vi "se_main.vi"(6 "se.mot.p.target":cluster{"x":fxp<+/-,16,1>, "y":fxp<+/-,16,1>}, 8 "outputParams":T4, 9 "se.p.modes":T6, 10 "se.p.durationTrigger":u16=100, 11 "scanClocks":T7={"se.mot.p.clocks"={"moveToDecFactor"=0, "moveToWaveSize"=0, "se.mot.p.invDec"=0.0}, "se.p.clocks"={"outputRate"=0, "fastDecFactor"=0, "outWaveSizeFast"=0, "pplUpsampling"=0, "numLines"=0, "se.p.fastInvDec"=0.0, "se.p.slowUpStep"=0.0, "se.p.outWaveSizeSlow"=0, "blankingMax"=0, "se.p.fastBlanking"={"startFwd"=0, "endFwd"=0, "startBwd"=0, "endBwd"=0, "disableBlanking"=FALSE, "useCoarseCounter"=TRUE}}}) -> (0 "clocksOut":T3, 1 "se.o.position":T2 {"outputInt"."x" format="%.16g"; "outputInt"."y" format="%.16g"}, 2 "se.mot.s.origin":T5, 3 "se.mot.s.running":bool, 4 "indices":T1, 5 "debug":cluster{"blanking":u32, "pixelEvent":bool}, 7 "se.s.blankingOff":bool)   [LabVIEW 2016]
uses:
  <vilib>/rvi/Emulation/niFpgaEmulationIsFPGAContextNoSignature.vi
  <vilib>/rvi/Emulation/niFpgaSctlEmulationGetInTimedLoop.vi
  <vilib>/rvi/errors/niFpgaSetErrorForExecOnDevCompSimple.vi
  <vilib>/rvi/eio/common/nirviEmuReportErrorAndStop.vi
  <vilib>/rvi/DataTransferAndStorage/Container/Common/niFpgaContainerGetUniqueNameForEmu.vi
  <vilib>/rvi/FIFO/Fifo_Resource/nirvififoEmulationSetSize.vi
  <vilib>/rvi/FIFO/Fifo_Resource/nirviFifoEmulationQueueMgr.vi
  <instcachedir>/0/nirviFifoEmulationQueueMgr_E5CAEC123FF24DC58D834DCA3CDAA9B5.lvgen/nirviFifoEmulationQueueMgr_E5CAEC123FF24DC58D834DCA3CDAA9B5_010.vi
  <vilib>/rvi/FIFO/Fifo_Resource/nirvififoEmulationDetermineInputValidOut.vi
  <vilib>/rvi/FIFO/Fifo_Resource/nirvififoEmulationCreateLock.vi
  <vilib>/rvi/Emulation/niFpgaProcessEmulError.vi
  <vilib>/rvi/FIFO/Fifo_Resource/nirvififoEmulationObtainLock.vi
  <vilib>/rvi/FIFO/Fifo_Resource/nirvififoEmulationReleaseLock.vi
  <vilib>/rvi/occurrence/nirviWaitOnOccurrenceBase.vi
  <vilib>/rvi/errors/nirviReportUnexpectedCaseInternalError.vi
  <vilib>/rvi/errors/nirviReportUnexpectedCaseInternalError (U32).vi
  <vilib>/rvi/Memory/Memory_Emulation/niFpgaMemoryEmulationCacheClearOnFirstRun.vi
  <vilib>/rvi/Memory/Memory_Emulation/nirvimemoryEmulationManagerCache_MakeExclusive.vi
  <vilib>/rvi/Memory/Memory_Emulation/niFpgaMemoryEmulationValidateCache.vi
  <vilib>/rvi/Memory/Memory_Emulation/nirvimemoryEmulationManagerCache_InsertValue.vi
  <vilib>/Utility/error.llb/Clear Errors.vi
  <vilib>/rvi/Memory/Memory_Emulation/nirvimemoryEmulationManagerCache_ReleaseExclusive.vi
  <vilib>/rvi/Memory/Memory_Emulation/nirvimemoryEmulationManagerCache_GetValue.vi
  <vilib>/rvi/Memory/Memory_Emulation/nirvimemoryEmulationManagerCache_SetValue.vi
  <vilib>/rvi/DataTransferAndStorage/Container/XNode/niFpgaContainer.xnode
  <vilib>/rvi/FIFO/Fifo_Resource/nirvififoEmulationWrite.vi
  <vilib>/rvi/DataTransferAndStorage/Register/Emulation/niFpgaRegisterEmulation.vi
  <vilib>/rvi/FXPMathLib/FxpInterpret/XNode/nifxpmath_Interpret.xnode
  <instrlib>/_niInstr/Basic Elements/v1/FPGA/niInstr Basic Elements v1 FPGA.lvlib
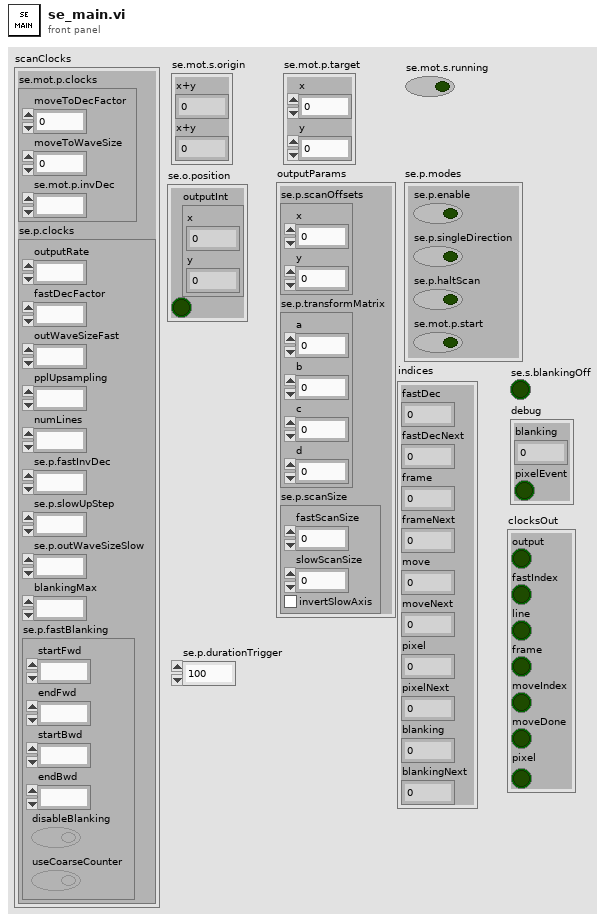
[diagram p1: front panel]
types:
  T1 = cluster{"fastDec":u16, "fastDecNext":u16, "frame":u16, "frameNext":u16, "move":u16, "moveNext":u16, "pixel":u16, "pixelNext":u16, "blanking":u32, "blankingNext":u32}
  T2 = cluster{"outputInt":cluster{"y":fxp<+/-,16,1>, "y":fxp<+/-,16,1>}, bool}
  T3 = cluster{"output":bool, "fastIndex":bool, "line":bool, "frame":bool, "moveIndex":bool, "moveDone":bool, "pixel":bool}
  T4 = cluster{"se.p.scanOffsets":cluster{"x":fxp<+/-,16,1>, "y":fxp<+/-,16,1>}, "se.p.transformMatrix":cluster{"a":fxp<+/-,18,2>, "b":fxp<+/-,18,2>, "c":fxp<+/-,18,2>, "d":fxp<+/-,18,2>}, "se.p.scanSize":cluster{"fastScanSize":fxp<+,17,1>, "slowScanSize":fxp<+,17,1>, "invertSlowAxis":bool}}
  T5 = cluster{"x+y":fxp<+/-,18,2>, "x+y":fxp<+/-,18,2>}
  T6 = cluster{"se.p.enable":bool, "se.p.singleDirection":bool, "se.p.haltScan":bool, "se.mot.p.start":bool}
  T7 = cluster{"se.mot.p.clocks":cluster{"moveToDecFactor":u16, "moveToWaveSize":u16, "se.mot.p.invDec":fxp<+,16,0>}, "se.p.clocks":cluster{"outputRate":u16, "fastDecFactor":u16, "outWaveSizeFast":u16, "pplUpsampling":u16, "numLines":u16, "se.p.fastInvDec":fxp<+,22,0>, "se.p.slowUpStep":fxp<+,28,0>, "se.p.outWaveSizeSlow":u16, "blankingMax":u32, "se.p.fastBlanking":cluster{"startFwd":u32, "endFwd":u32, "startBwd":u32, "endBwd":u32, "disableBlanking":bool, "useCoarseCounter":bool}}}
  T8 = cluster{"moveToDecFactor":u16, "moveToWaveSize":u16, "se.mot.p.invDec":fxp<+,16,0>}
  T9 = cluster{"outputRate":u16, "fastDecFactor":u16, "outWaveSizeFast":u16, "pplUpsampling":u16, "numLines":u16, "se.p.fastInvDec":fxp<+,22,0>, "se.p.slowUpStep":fxp<+,28,0>, "se.p.outWaveSizeSlow":u16, "blankingMax":u32, "se.p.fastBlanking":cluster{"startFwd":u32, "endFwd":u32, "startBwd":u32, "endBwd":u32, "disableBlanking":bool, "useCoarseCounter":bool}}
  T10 = cluster{"startFwd":u32, "endFwd":u32, "startBwd":u32, "endBwd":u32, "disableBlanking":bool, "useCoarseCounter":bool}
  T11 = cluster{"index":u16, "next":u16, "blanking":u32, "blankingNext":u32}
  T12 = cluster{"interpOutput":fxp<+/-,19,2>, "interpOutput":fxp<+/-,19,2>}
  T13 = cluster{"a":fxp<+/-,18,2>, "b":fxp<+/-,18,2>, "c":fxp<+/-,18,2>, "d":fxp<+/-,18,2>}
  T14 = cluster{"fastScanSize":fxp<+,17,1>, "slowScanSize":fxp<+,17,1>, "invertSlowAxis":bool}
  T15 = cluster{"se.p.scanOffsets":cluster{"x":bool, "y":bool}, "se.p.transformMatrix":cluster{"a":bool, "b":bool, "c":bool, "d":bool}, "se.p.scanSize":cluster{"fastScanSize":bool, "slowScanSize":bool, "invertSlowAxis":bool}}
  T16 = cluster{"xOut":fxp<+/-,18,2>, "yOut":fxp<+/-,18,2>}
  T17 = cluster{"fastScanSize":bool, "slowScanSize":bool, "invertSlowAxis":bool}
  T18 = cluster{cluster{"y":fxp<+/-,16,1>, "y":fxp<+/-,16,1>}, bool}
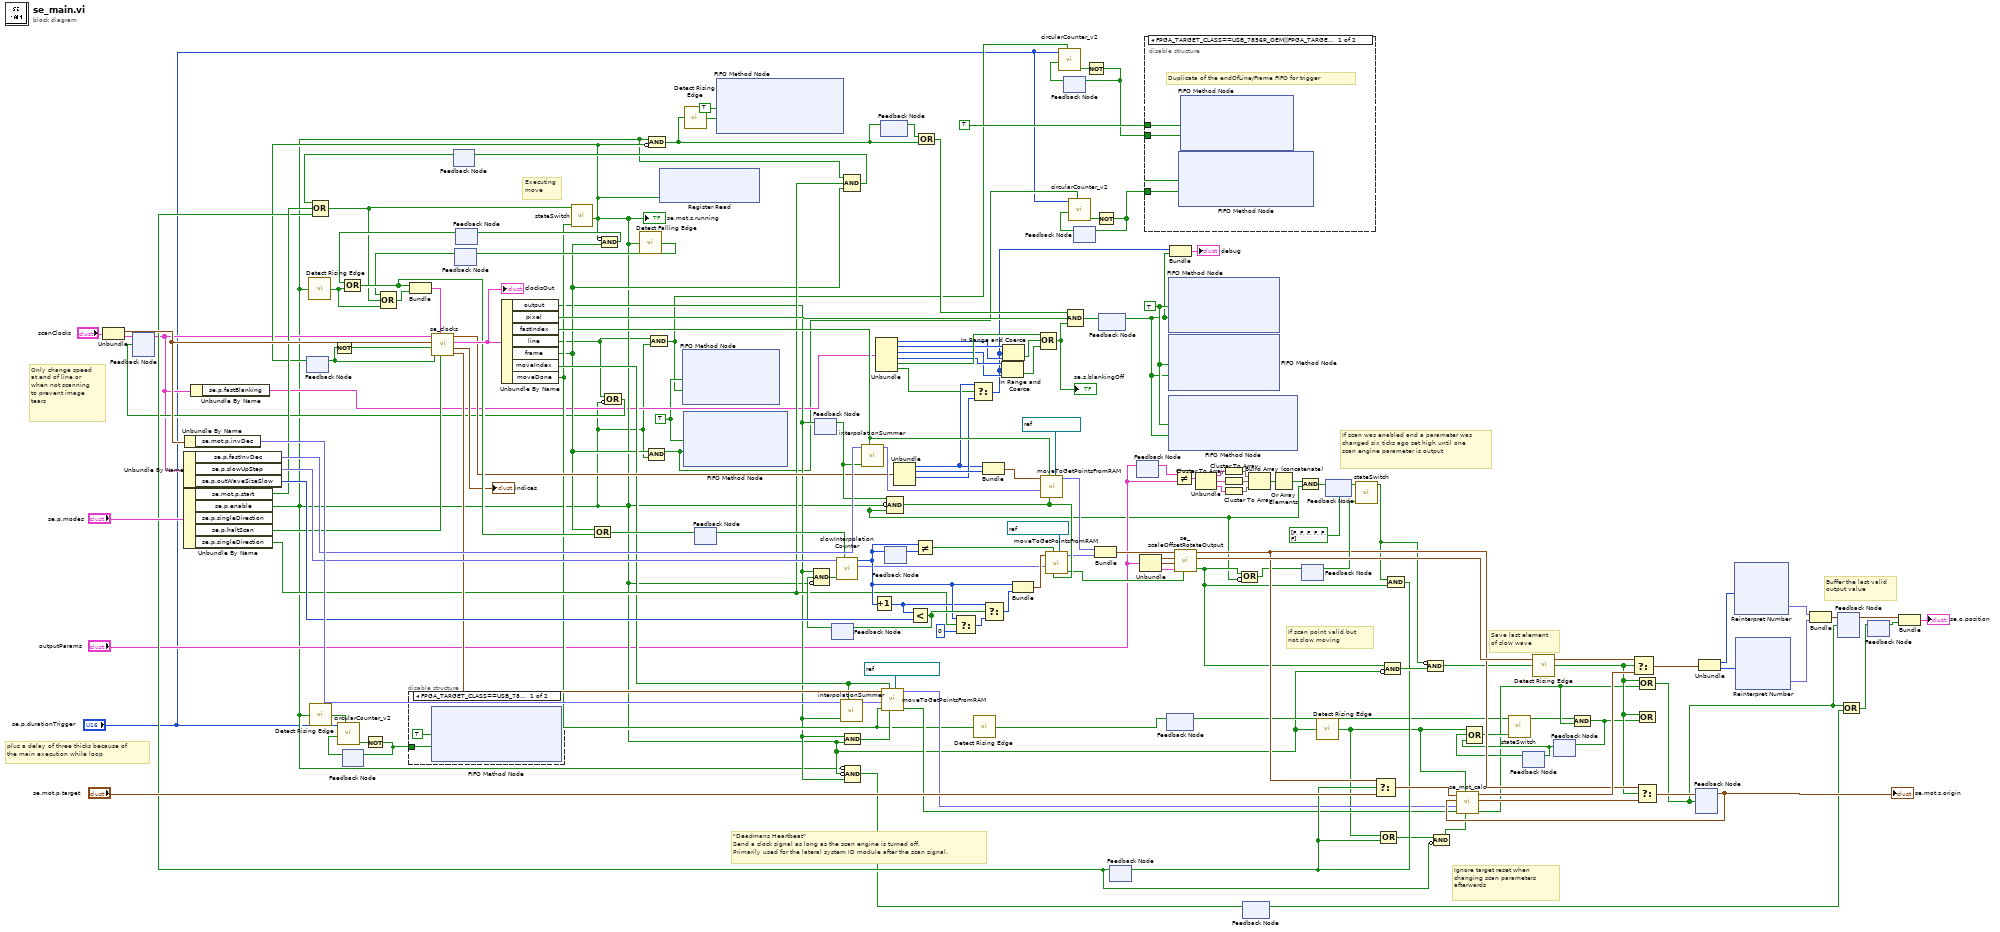
[diagram p0: block diagram]
diagram:
  w2 = TRUE ("Element")
  w20 = TRUE ("Element")
  # "plus a delay of three thicks because of\nthe main execution while loop"
  # "Only change speed at end of line or when not scanning to prevent image tears"
  # "Buffer the last valid output value"
  # "\"Deadmans Heartbeat\"\nSend a clock signal as long as the scan engine is turned off.\nPrimarily used for the lateral system ID module after the scan signal."
  # "Ignore target reset when changing scan parameters afterwards"
  # "If scan point valid but not slow moving"
  # "If scan was enabled and a parameter was changed six ticks ago set high until one scan engine parameter is output"
  # "Save last element \nof slow wave"
  # "Executing\nmove"
  n1 = Unbundle("scanClocks") -> ("se.mot.p.clocks"=w164:T8, "se.p.clocks"=w25:T9)
  n2 = feedback #1() -> (w24:T9)  [unwired: 1 in]
  n3 = Unbundle By Name(w24) -> ("se.p.fastInvDec"=w159:fxp<+,22,0>, "se.p.slowUpStep"=w160:fxp<+,28,0>, "se.p.outWaveSizeSlow"=w161:u16)
  n4 = Unbundle By Name("se.p.modes") -> ("se.mot.p.start"=w76:bool, "se.p.enable"=w14:bool, "se.p.haltScan"=w158:bool, "se.p.singleDirection"=w75:bool)  [unwired: 1 out]
  n5 = Unbundle By Name(w164) -> ("se.mot.p.invDec"=w162:fxp<+,16,0>)
  n6 = Unbundle By Name(w24) -> ("se.p.fastBlanking"=w26:T10)
  n7 = feedback #2() -> (w131:bool)  [unwired: 1 in]
  n8 = call <instrlib>:"Detect Rising Edge.vi"("signal"=w14) -> ("edge detected"=w74:bool)  [unwired: 14 in]
  n9 = call <instrlib>:"Detect Rising Edge.vi"("signal"=w14) -> ("edge detected"=w17:bool)  [unwired: 14 in]
  n10 = Not(x=w131) -> (.not. x?=w132:bool)
  n11 = feedback #3() -> (w15:bool)  [unwired: 1 in]
  n12 = call "circularCounter_v2.vi"("reset"=w17, "doStep"=w15, "maxCount"="se.p.durationTrigger") -> ("maxReached"=w18:bool)  [unwired: 5 in, 3 out]
  n13 = Not(x=w18) -> (.not. x?=w16:bool)
  n14 = feedback-in #3(w16) -> ()
  n15 = disable-structure shown="FPGA_TARGET_CLASS==USB_7856R_OEM||FPGA_TARGET_CLASS==USB_7856R" {
    disable-tunnel: w16 -> [w165 _]
    frame condition #0 (active) {
      n16 = xnode ("FIFO Method Node")("Element"=TRUE, "Input Valid"=w165) -> ()  [unwired: 1 in, 2 out]
    }
    frame condition #1 {
    }
  }
  n17 = feedback #4() -> (w127:bool)  [unwired: 1 in]
  n18 = feedback #5() -> (w72:bool)  [unwired: 1 in]
  n19 = feedback #6() -> (w124:bool)  [unwired: 1 in]
  n20 = Compound Arithmetic op=OR(w124, w74) -> (w91:bool)
  n21 = feedback #7() -> (w136:bool)  [unwired: 1 in]
  n22 = feedback #8() -> (w137:bool)  [unwired: 1 in]
  n23 = feedback #9() -> (w135:bool)  [unwired: 1 in]
  n24 = Unbundle(w26) -> ("startFwd"=w143:u32, "endFwd"=w144:u32, "startBwd"=w145:u32, "endBwd"=w146:u32, "disableBlanking"=w149:bool, "useCoarseCounter"=w64:bool)
  n25 = feedback #10() -> (w139:bool)  [unwired: 1 in]
  n26 = feedback #11() -> (w121:u16)  [unwired: 1 in]
  n27 = feedback #12() -> (w13:bool)  [unwired: 1 in]
  n28 = feedback #13() -> (w8:bool)  [unwired: 1 in]
  n29 = feedback #14() -> (w1:bool)  [unwired: 1 in]
  n30 = feedback #15() -> (w45:bool)  [unwired: 1 in]
  n31 = Compound Arithmetic op=OR(w127, w76, w45) -> (w73:bool)
  n32 = Compound Arithmetic op=OR(w72, w73, w74) -> (w89:bool)
  n33 = Bundle(w91, w89) -> (w90:cluster{bool, bool})  [unwired: 1 in]
  n34 = call "se_clocks.vi"("haltScan"=w158, "se.p.resetClocks"=w90, "stepSlow"=w131, "stepScan"=w132, "moveRates"=w164, "se.p.clocks"=w24) -> ("moveIndices"=w87:cluster{"index":u16, "next":u16}, "indices"=→"indices":T1, "clocks"=w117:T3, "fastIndices"=w88:T11)  [unwired: 2 in]
  "clocksOut" <- w117
  n35 = Unbundle By Name(w117) -> ("output"=w38:bool, "pixel"=w138:bool, "fastIndex"=w119:bool, "line"=w28:bool, "frame"=w44:bool, "moveIndex"=w58:bool, "moveDone"=w53:bool)
  n36 = call "stateSwitch.vi"("disable"=w53, "enable"=w73) -> ("state"=w37:bool)  [unwired: 9 in]
  "se.mot.s.running" <- w37
  n37 = feedback-in #2(w37) -> ()
  n38 = Compound Arithmetic op=OR(w44, w91) -> (w128:bool)
  n39 = Compound Arithmetic op=AND(invert w37, w44) -> (w130:bool)
  n40 = feedback-in #6(w130) -> ()
  n41 = Compound Arithmetic op=OR(w28, invert w14) -> (w27:bool)
  n42 = feedback-in #1(w25, w27) -> ()
  n43 = call <instrlib>:"Detect Falling Edge.vi"("signal"=w37) -> ("edge detected"=w129:bool)  [unwired: 14 in]
  n44 = feedback-in #5(w129) -> ()
  n45 = Compound Arithmetic op=AND(w44, w14) -> (w7:bool)
  n46 = Compound Arithmetic op=AND(w14, invert w37) -> (w140:bool)
  n47 = Compound Arithmetic op=AND(w28, w14) -> (w11:bool)
  n48 = xnode ("Register Read")("Data"=w37) -> ()  [unwired: 1 in, 1 out]
  n49 = xnode ("FIFO Method Node")("Element"=w20, "Input Valid"=w11) -> ()  [unwired: 1 in, 2 out]
  n50 = xnode ("FIFO Method Node")("Element"=w20, "Input Valid"=w7) -> ()  [unwired: 1 in, 2 out]
  n51 = call <instrlib>:"Detect Rising Edge.vi"("signal"=w140) -> ("edge detected"=w4:bool)  [unwired: 14 in]
  n52 = feedback-in #7(w128) -> ()
  n53 = xnode ("FIFO Method Node")("Element"=TRUE, "Input Valid"=w4) -> ()  [unwired: 1 in, 2 out]
  n54 = Compound Arithmetic op=AND(w38, w135, invert w37) -> (w133:bool)
  n55 = feedback-in #8(w38) -> ()
  n56 = call "slowInterpolationCounter.vi"("reset"=w136, "doStep"=w133, "upStep"=w160) -> ("fraction"=w116:fxp<+,28,0>, "index"=w122:u16)  [unwired: 7 in]
  n57 = call "interpolationSummer.vi"("reset"=w58, "doStep"=w38, "upStep"=w162) -> ("position"=w106:fxp<+,22,0>)  [unwired: 8 in]
  n58 = Compound Arithmetic op=AND(w14, w75, w44) -> (w126:bool)
  n59 = feedback-in #4(w126) -> ()
  n60 = Compound Arithmetic op=AND(w38, w37) -> (w57:bool)
  n61 = Compound Arithmetic op=AND(invert w14, invert w37, w38) -> (w35:bool)
  n62 = call "interpolationSummer.vi"("reset"=w119, "doStep"=w137, "upStep"=w159) -> ("position"=w110:fxp<+,22,0>)  [unwired: 8 in]
  n63 = Increment(x=w122) -> (x+1=w107:u16)
  n64 = feedback-in #10(w140) -> ()
  n65 = call "moveToGetPointsFromRAM.vi"("Memory In"=refnum<k21> "se.mot.motion", "inputValid"=w57, "reset"=w58, "maxReached"=w53, "interpPosition"=w106, "adresses"=w87) -> ("outputValid"=w59:bool, "interpOutput"=w56:fxp<+/-,19,2>)  [unwired: 4 in]
  n66 = feedback-in #11(w122) -> ()
  n67 = Compound Arithmetic op=AND(w137, invert w37, w14) -> (w125:bool)
  n68 = Unbundle(w88) -> ("index"=w65:u16, "next"=w68:u16, "blanking"=w66:u32)  [unwired: 1 out]
  n69 = Less?(x=w107, y=w161) -> (x < y?=w134:bool)
  n70 = feedback-in #9(w134) -> ()
  n71 = Not Equal?(x=w122, y=w121) -> (x != y?=w123:bool)
  n72 = Compound Arithmetic op=OR(w139, w140) -> (w141:bool)
  n73 = Select(t=w122, s=w75, f=u16 0) -> (s? t:f=w108:u16)
  n74 = Select(t=w65, s=w64, f=w66) -> (s? t:f=w23:u32)
  n75 = call <instrlib>:"Detect Rising Edge.vi"("signal"=w53) -> ("edge detected"=w49:bool)  [unwired: 14 in]
  n76 = Bundle("index"=w65, "next"=w68) -> (w67:cluster{"index":u16, "next":u16})  [unwired: 1 in]
  n77 = Select(t=w107, s=w134, f=w108) -> (s? t:f=w115:u16)
  n78 = In Range and Coerce(upper limit=w146, x=w23, lower limit=w145) -> (In Range?=w147:bool)  [unwired: 1 out]
  n79 = In Range and Coerce(upper limit=w144, x=w23, lower limit=w143) -> (In Range?=w148:bool)  [unwired: 1 out]
  n80 = Bundle("index"=w122, "f"=w115) -> (w120:cluster{"index":u16, "f":u16})  [unwired: 1 in]
  n81 = Compound Arithmetic op=OR(w149, w148, w147) -> (w142:bool)
  "se.s.blankingOff" <- w142
  n82 = call "moveToGetPointsFromRAM.vi"("Memory In"=refnum<k21> "se.fastAxis", "inputValid"=w125, "reset"=w119, "interpPosition"=w110, "adresses"=w67) -> ("interpOutput"=w112:fxp<+/-,19,2>)  [unwired: 5 in, 1 out]
  n83 = call "moveToGetPointsFromRAM.vi"("Memory In"=refnum<k21> "se.slowAxis", "inputValid"=w125, "reset"=w123, "interpPosition"=w116, "adresses"=w120) -> ("outputValid"=w80:bool, "interpOutput"=w113:fxp<+/-,19,2>)  [unwired: 5 in]
  n84 = call "circularCounter_v2.vi"("reset"=w11, "doStep"=w13, "maxCount"="se.p.durationTrigger") -> ("maxReached"=w12:bool)  [unwired: 5 in, 3 out]
  n85 = Compound Arithmetic op=AND(w141, w138, w142) -> (w21:bool)
  n86 = call "circularCounter_v2.vi"("reset"=w7, "doStep"=w8, "maxCount"="se.p.durationTrigger") -> ("maxReached"=w9:bool)  [unwired: 5 in, 3 out]
  n87 = Not(x=w12) -> (.not. x?=w10:bool)
  n88 = feedback-in #12(w10) -> ()
  n89 = Bundle("interpOutput"=w112, "interpOutput"=w113) -> (w114:T12)  [unwired: 1 in]
  n90 = Not(x=w9) -> (.not. x?=w6:bool)
  n91 = feedback-in #13(w6) -> ()
  n92 = feedback-in #14(w21) -> ()
  n93 = feedback-in #16("outputParams") -> ()
  n94 = feedback #16() -> (w104:T4)  [unwired: 1 in]
  n95 = Unbundle("outputParams") -> ("se.p.scanOffsets"=w150:cluster{"x":fxp<+/-,16,1>, "y":fxp<+/-,16,1>}, "se.p.transformMatrix"=w151:T13, "se.p.scanSize"=w152:T14)
  n96 = disable-structure shown="FPGA_TARGET_CLASS==USB_7856R_OEM||FPGA_TARGET_CLASS==USB_7856R" {
    disable-tunnel: TRUE ("Input Valid") -> [w169 _]
    disable-tunnel: w10 -> [w168 _]
    disable-tunnel: w6 -> [w167 _]
    frame condition #0 (active) {
      # "Duplicata of the endOfLine/Frame FIFO for trigger"
      n97 = xnode ("FIFO Method Node")("Element"=w169, "Input Valid"=w167) -> ()  [unwired: 1 in, 2 out]
      n98 = xnode ("FIFO Method Node")("Element"=w169, "Input Valid"=w168) -> ()  [unwired: 1 in, 2 out]
    }
    frame condition #1 {
    }
  }
  n99 = feedback #17() -> (w48:bool)  [unwired: 1 in]
  n100 = feedback-in #17(w49) -> ()
  n101 = xnode ("FIFO Method Node")("Element"=w2, "Input Valid"=w1) -> ()  [unwired: 1 in, 2 out]
  n102 = xnode ("FIFO Method Node")("Element"=w2, "Input Valid"=w1) -> ()  [unwired: 1 in, 2 out]
  n103 = xnode ("FIFO Method Node")("Element"=w2, "Input Valid"=w1) -> ()  [unwired: 1 in, 2 out]
  n104 = Bundle("blanking"=w23, w1) -> (→"debug":cluster{"blanking":u32, bool})  [unwired: 1 in]
  n105 = Not Equal?(x=w104, y="outputParams") -> (x != y?=w103:T15)
  n106 = call "se_scaleOffsetRotateOutput.vi"("inputValid"=w80, "scanSize"=w152, "outputMatrix"=w151, "scanOffset"=w150, "input"=w114) -> ("outputValid"=w51:bool, "outputInt"=w156:cluster{"x":i16, "y":i16}, "outputNorm"=w93:T16)  [unwired: 4 in]
  n107 = Unbundle(w103) -> ("se.p.scanOffsets"=w102:cluster{"x":bool, "y":bool}, "se.p.transformMatrix"=w101:cluster{"a":bool, "b":bool, "c":bool, "d":bool}, "se.p.scanSize"=w100:T17)
  n108 = Cluster To Array(cluster=w102) -> (array=w99:bool[])
  n109 = Cluster To Array(cluster=w101) -> (array=w98:bool[])
  n110 = Cluster To Array(cluster=w100) -> (array=w97:bool[])
  n111 = Compound Arithmetic op=OR(w51, invert w14) -> (w50:bool)
  n112 = feedback #18() -> (w34:bool)  [unwired: 1 in]
  n113 = feedback-in #18(w35) -> ()
  n114 = Build Array (concatenate)(w99, w98, w97) -> (w96:bool[])
  n115 = Or Array Elements(Boolean array=w96) -> (logical OR=w95:bool)
  n116 = feedback #19() -> (w94:bool)  [unwired: 1 in]
  n117 = feedback-in #19(w50) -> ()
  n118 = Compound Arithmetic op=AND(w95, w14) -> (w78:bool)
  n119 = call <instrlib>:"Detect Rising Edge.vi"("signal"=w37) -> ("edge detected"=w47:bool)  [unwired: 14 in]
  n120 = feedback-in #20(w78) -> ()
  n121 = feedback #20(bool[] [FALSE, FALSE, FALSE, FALSE, FALSE, FALSE]) -> (w83:bool)
  n122 = call "stateSwitch.vi"("disable"=w94, "enable"=w83) -> ("state"=w60:bool)  [unwired: 9 in]
  n123 = Compound Arithmetic op=AND(w51, invert w37) -> (w79:bool)
  n124 = Compound Arithmetic op=AND(w60, w51) -> (w61:bool)
  n125 = feedback-in #15(w61) -> ()
  n126 = Select(t=w93, s=w61, f="se.mot.p.target") -> (s? t:f=w84:T16)
  n127 = Compound Arithmetic op=OR(w47, w61) -> (w52:bool)
  n128 = Compound Arithmetic op=AND(invert w60, w79) -> (w62:bool)
  n129 = Compound Arithmetic op=AND(w52, invert w45) -> (w46:bool)
  n130 = feedback #21() -> (w69:bool)  [unwired: 1 in]
  n131 = call <instrlib>:"Detect Rising Edge.vi"("signal"=w62) -> ("edge detected"=w82:bool)  [unwired: 14 in]
  n132 = feedback #22() -> (w70:bool)  [unwired: 1 in]
  n133 = Compound Arithmetic op=OR(w47, w69, w70) -> (w71:bool)
  n134 = call "stateSwitch.vi"("disable"=w71, "enable"=w48) -> ("state"=w54:bool)  [unwired: 9 in]
  n135 = feedback-in #21(w70) -> ()
  n136 = feedback #23() -> (w85:T5)  [unwired: 1 in]
  "se.mot.s.origin" <- w85
  n137 = call "se_mot_calc.vi"("targetValid"=w46, "resetOrigin"=w47, "inputValid"=w59, "interpOutput"=w56, "origin"=w85, "se.mot.p.target"=w84) -> ("outputValid"=w55:bool, "outputNorm"=w154:T5, "outputInt"=w153:cluster{"x":i16, "y":i16})  [unwired: 3 in]
  n138 = Compound Arithmetic op=AND(w54, w55) -> (w81:bool)
  n139 = feedback-in #22(w81) -> ()
  n140 = Select(t=w156, s=w82, f=w153) -> (s? t:f=w43:cluster{"x":i16, "y":i16})
  n141 = Select(t=w93, s=w82, f=w154) -> (s? t:f=w63:T5)
  n142 = Compound Arithmetic op=OR(w82, w55) -> (w31:bool)
  n143 = Compound Arithmetic op=OR(w82, w81) -> ()  [unwired: 1 out]
  n144 = feedback-in #23(w63, w31) -> ()
  n145 = Unbundle(w43) -> ("x"=w42:i16, "y"=w41:i16)
  n146 = xnode "Reinterpret Number"("x"=w42) -> ("y"=w40:fxp<+/-,16,1>)
  n147 = xnode "Reinterpret Number"("x"=w41) -> ("y"=w39:fxp<+/-,16,1>)
  n148 = Bundle("y"=w40, "y"=w39) -> (w33:cluster{"y":fxp<+/-,16,1>, "y":fxp<+/-,16,1>})  [unwired: 1 in]
  n149 = feedback-in #24(w33, w31) -> ()
  n150 = feedback #24() -> (w32:cluster{"y":fxp<+/-,16,1>, "y":fxp<+/-,16,1>})  [unwired: 1 in]
  n151 = Compound Arithmetic op=OR(w31, w34) -> (w36:bool)
  n152 = feedback-in #25(w36) -> ()
  n153 = feedback #25() -> (w30:bool)  [unwired: 1 in]
  n154 = Bundle(w32, w30) -> (→"se.o.position":T18)  [unwired: 1 in]
